vi "Handle Events.vi"(8 "error in (no error)":errorcluster, 11 "ControlEventHandler":refnum<class "ControlEventHandler.lvclass">) -> ()   [LabVIEW 2015, in "ActorEvents.lvlib" / "ControlEventHandler.lvclass"]
uses:
  ControlEventHandler.lvclass
  IEventHandler/IEventHandler.lvclass/IEventHandler.ctl
  ControlEventHandler.lvclass/ControlEventHandler.ctl
  <vilib>/ActorFramework/Message Enqueuer/Message Enqueuer.lvclass/Message Enqueuer.ctl
  <vilib>/ActorFramework/Message Priority Queue/Priority Enqueue.vi
  IEventHandler/IEventHandler.lvclass
  ActorAutoRegistration Messages/ValueChangeMsg/ValueChangeMsg.lvclass
  ActorAutoRegistration Messages/ControlMouseDownMsg/ControlMouseDownMsg.lvclass
  ActorAutoRegistration Messages/ControlMouseUpMsg/ControlMouseUpMsg.lvclass
  <vilib>/ActorFramework/Message Enqueuer/Message Enqueuer.lvclass
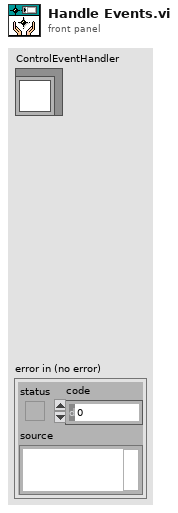
[diagram p1: front panel]
types:
  T1 = typedef "Actor Framework.lvlib/Message Enqueuer.lvclass/Message Priority.ctl" = enum16{"Low", "Normal", "High"}
  T2 = typedef "LVPoint32TypeDef.ctl" = cluster{"Horizontal":i32, "Vertical":i32}
  T3 = cluster{"Shift":bool, "Ctrl":bool, "Alt":bool, "Cmd":bool, "Opt":bool}
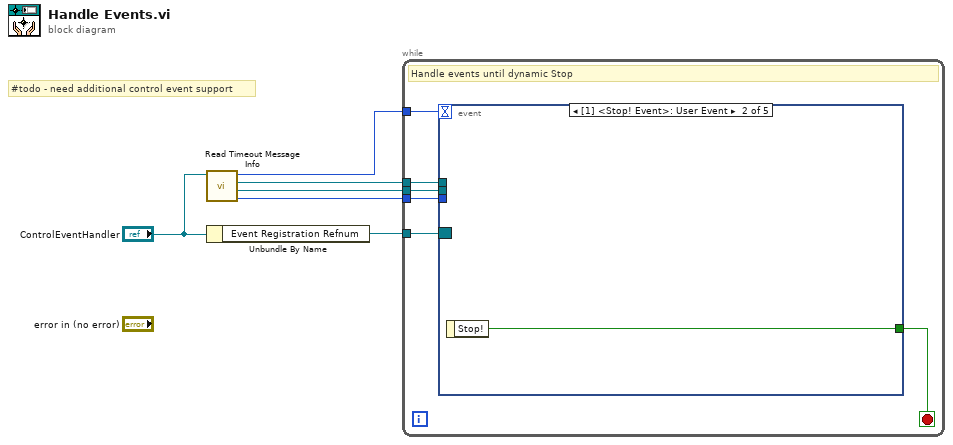
[diagram p0: block diagram]
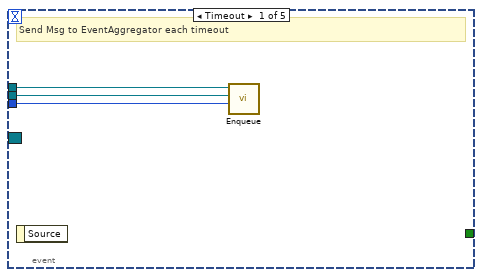
[diagram p2: hidden frame]
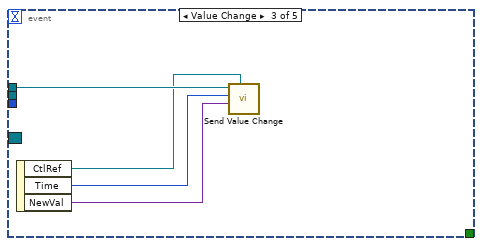
[diagram p3: hidden frame]
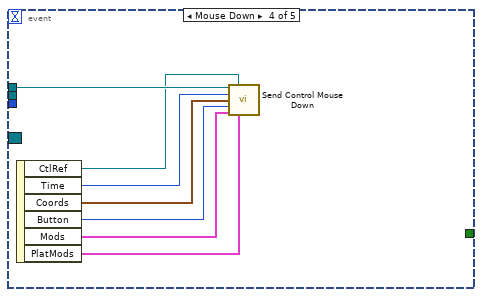
[diagram p4: hidden frame]
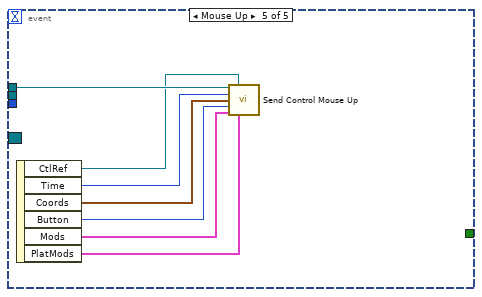
[diagram p5: hidden frame]
diagram:
  # "#todo - need additional control event support"
  n1 = call "Read Timeout Message Info.vi"("IEventHandler in"="ControlEventHandler") -> ("Timeout Message Priority"=w2:T1, "Timeout Message"=w3:refnum<class "Message.lvclass">, "EventAggregator Enqueuer"=w4:refnum<class "Message Enqueuer.lvclass">, "Timeout [ms]"=w1:i32)  [unwired: 7 in]
  n2 = Unbundle By Name("ControlEventHandler") -> ("Event Registration Refnum"=w6:refnum<event-registration>)
  n3 = while {
    tunnel: w6 -> [w12]
    tunnel: w4 -> [w10]
    tunnel: w3 -> [w9]
    tunnel: w2 -> [w8]
    tunnel: w1 -> [w7]
    stop <- w11 stop-if-true
    # "Handle events until dynamic Stop"
    n4 = event shown="[1] <Stop! Event>: User Event" {
      selector: w12 -> [_ _ _ _ _]
      dyn-events: _ -> [_ _ _ _ _]
      timeout: w7 -> [_ _ _ _ _]
      tunnel: [_ w16 _ _ _] -> w11
      tunnel: w10 -> [w15 _ w20 w27 w34]
      tunnel: w9 -> [w14 _ _ _ _]
      tunnel: w8 -> [w13 _ _ _ _]
      event Timeout {
        # "Send Msg to EventAggregator each timeout"
        n5 = event-data() -> ()  [unwired: 1 in, 1 out]
        n6 = call <vilib>:"Enqueue.vi"("Message Priority (Normal)"=w13, "Message"=w14, "Message Enqueuer in"=w15) -> ()  [unwired: 7 in, 2 out]
      }
      event User Event {
        n7 = event-data() -> ("Stop!"=w16:bool)  [unwired: 1 in]
      }
      event Value Change {
        n8 = event-data() -> ("CtlRef"=w17:refnum<vi>, "Time"=w19:u32, "NewVal"=w18:variant)  [unwired: 1 in]
        n9 = call "Send Value Change.vi"("Ctl Refnum"=w17, "New Value"=w18, "Time"=w19, "Message Enqueuer in"=w20) -> ()  [unwired: 7 in, 1 out]
      }
      event Mouse Down {
        n10 = event-data() -> ("CtlRef"=w25:refnum<vi>, "Time"=w26:u32, "Coords"=w24:T2, "Button"=w23:u16, "Mods"=w22:cluster{"Double Click":bool, "Menu Key":bool}, "PlatMods"=w21:T3)  [unwired: 1 in]
        n11 = call "Send Control Mouse Down.vi"("Message Enqueuer in"=w27, "Ctl Refnum"=w25, "Time"=w26, "Coords"=w24, "Button"=w23, "Mods"=w22, "PlatMods"=w21) -> ()  [unwired: 8 in, 1 out]
      }
      event Mouse Up {
        n12 = event-data() -> ("CtlRef"=w32:refnum<vi>, "Time"=w33:u32, "Coords"=w31:T2, "Button"=w30:u16, "Mods"=w29:cluster{"Double Click":bool, "Menu Key":bool}, "PlatMods"=w28:T3)  [unwired: 1 in]
        n13 = call "Send Control Mouse Up.vi"("Message Enqueuer in"=w34, "Ctl Refnum"=w32, "Time"=w33, "Coords"=w31, "Button"=w30, "Mods"=w29, "PlatMods"=w28) -> ()  [unwired: 8 in, 1 out]
      }
    }
  }
